vi "Digitizer Fail Warning.vi"(8 "ATS Ref":string, 9 "Scope Address":refnum<visa-resource-name>="HDO9404", 10 "Digitizer Config":i32(ring)=4 items=["Single channel", "2 Chans w/ 2 Acqiris", "2 Chans w/ 1 Acqiris", "5-CH Pulser New", "5-CH pulser w/ ann array", "5-pass style ann array", "Empty"], 11 "Main Digitizer":T1=enum."NI Digitizer") -> (0 "Retry":bool, 1 "Scope Address":refnum<visa-resource-name>, 2 "Digitizer Config":i32(ring)=4 items=["Single channel"=0, "2 Chans w/ 2 Acqiris"=1, "2 Chans w/ 1 Acqiris"=2, "5-CH pulser w/ ann array"=4, "5-pass style ann array"=5], 3 "Main Digitizer":T1=enum."NI Digitizer", 4 "ATS Ref":string)   [LabVIEW 2022 SP3]
uses:
  Digitizer.ctl
panel:
  in  "Ignore":bool
  in  "Abort":bool
  in  "Try Again":bool
  # "Digitizer Initialization Failed!"
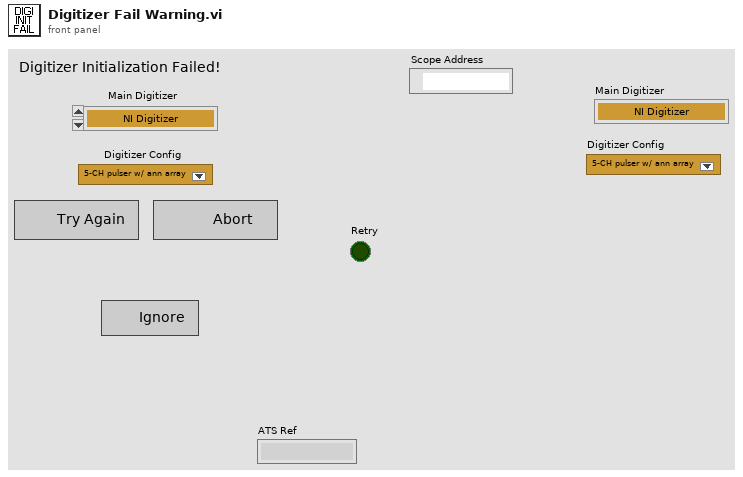
[diagram p1: front panel]
types:
  T1 = typedef "Digitizer.ctl" = enum16{"Acqiris Digitizer", "NI Digitizer", "LeCroy", "GaGe", "AlazarTech", "No Digitizer", "Teledyne"}
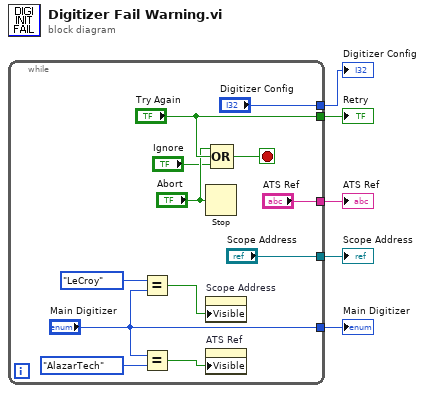
[diagram p0: block diagram]
diagram:
  n1 = while {
    tunnel: ["Main Digitizer"] -> w5
    tunnel: ["Digitizer Config"] -> w4
    tunnel: ["Try Again"] -> w3
    tunnel: ["Scope Address"] -> w2
    tunnel: ["ATS Ref"] -> w1
    stop <- w16 stop-if-true
    n2 = Equal?(x=Digitizer."LeCroy", y="Main Digitizer") -> (x = y?=w12:bool)
    n3 = Equal?(x="Main Digitizer", y=Digitizer."AlazarTech") -> (x = y?=w8:bool)
    n4 = Stop(stop? (T)="Abort") -> ()
    n5 = property on="Scope Address" class="VISAName"("Visible"=w12) -> ()  [unwired: 2 in, 2 out]
    n6 = property on="ATS Ref" class="Str"("Visible"=w8) -> ()  [unwired: 2 in, 2 out]
    n7 = Compound Arithmetic op=OR("Abort", "Try Again", "Ignore") -> (w16:bool)
  }
  "Main Digitizer" <- w5
  "Digitizer Config" <- w4
  "Retry" <- w3
  "Scope Address" <- w2
  "ATS Ref" <- w1
